vi "VHardCopy.vi"(8 "error in (no error)":errorcluster, 9 "File path":string="Z:\\DSOS404", 10 "TimeStamp":string="201711091540DSO404", 11 "VISA resource name":refnum<visa-resource-name>="DSOS404") -> (0 "error out":errorcluster, 3 "VISA resource name out":refnum<visa-resource-name>)   [LabVIEW 2018]
panel:
  out "concatenated string":string
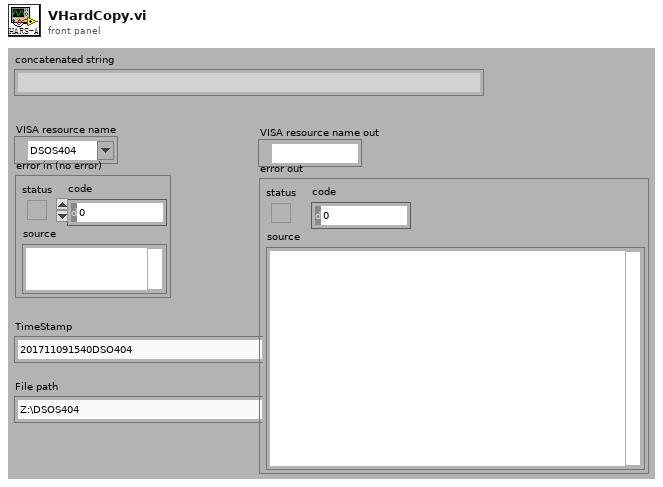
[diagram p1: front panel]
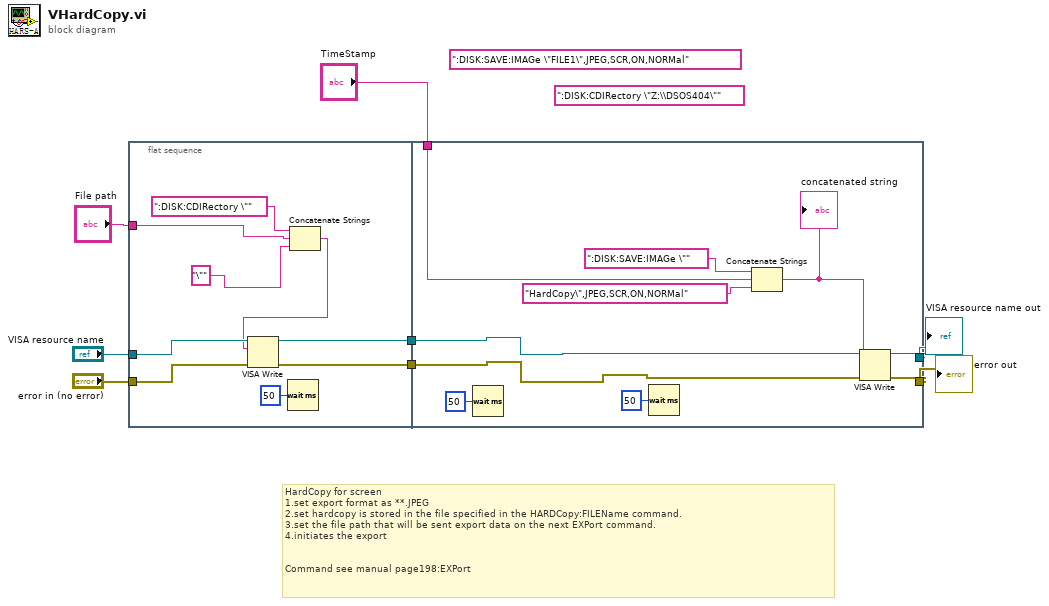
[diagram p0: block diagram]
diagram:
  (unwired) ":DISK:CDIRectory \"Z:\\DSOS404\"" ("write buffer")
  (unwired) ":DISK:SAVE:IMAGe \"FILE1\",JPEG,SCR,ON,NORMal" ("write buffer")
  # "HardCopy for screen\n1.set export format as **.JPEG\n2.set hardcopy is stored in the file specified in the HARDCopy:FILEName command. \n3.set the file path that will be sent export data on the next EXPort command.\n4.initiates the export\n\n\nCommand see manual page198:EXPort"
  n1 = flat-sequence {
    tunnel: "File path" -> [w9]
    tunnel: "error in (no error)" -> [w16]
    tunnel: "VISA resource name" -> [w17]
    tunnel: [w15] -> w3
    tunnel: [w14] -> w2
    tunnel: [w18] -> w4
    tunnel: [w19] -> w5
    tunnel: "TimeStamp" -> [w21]
    tunnel: w3 -> [w23]
    tunnel: w2 -> [w22]
    frame #0 {
      n2 = Wait (ms)(milliseconds to wait=u32 50) -> ()  [unwired: 1 out]
      n3 = Concatenate Strings(":DISK:CDIRectory \"" ("write buffer"), w9, "\"" ("format string")) -> (w11:string)
      n4 = VISA Write(VISA resource name=w17, write buffer=w11, error in (no error)=w16) -> (VISA resource name out=w15:refnum<visa-resource-name>, error out=w14:errorcluster)  [unwired: 1 out]
    }
    frame #1 {
      n5 = Wait (ms)(milliseconds to wait=u32 50) -> ()  [unwired: 1 out]
      n6 = Wait (ms)(milliseconds to wait=u32 50) -> ()  [unwired: 1 out]
      n7 = Concatenate Strings(":DISK:SAVE:IMAGe \"" ("write buffer"), w21, "HardCopy\",JPEG,SCR,ON,NORMal" ("format string")) -> (w26:string)
      "concatenated string" <- w26
      n8 = VISA Write(VISA resource name=w23, write buffer=w26, error in (no error)=w22) -> (VISA resource name out=w19:refnum<visa-resource-name>, error out=w18:errorcluster)  [unwired: 1 out]
    }
  }
  "VISA resource name out" <- w5
  "error out" <- w4
